vi "1 sample delay 8spc.vi"(8 "input valid":bool=TRUE, 10 "delay":u8, 11 "IQ in":T1(array[cluster])=[{"I"=0.0, "Q"=0.0, "overflow"=FALSE}, {"I"=0.0, "Q"=0.0, "overflow"=FALSE}, {"I"=0.0, "Q"=0.0, "overflow"=FALSE}, {"I"=0.0, "Q"=0.0, "overflow"=FALSE}, {"I"=0.0, "Q"=0.0, "overflow"=FALSE}, {"I"=0.0, "Q"=0.0, "overflow"=FALSE}, {"I"=0.0, "Q"=0.0, "overflow"=FALSE}, {"I"=0.0, "Q"=0.0, "overflow"=FALSE}]) -> (0 "output valid":bool, 3 "IQ out":T1(array[cluster]))   [LabVIEW 2021]
doc: "sum 2 IQ datas (I+I =>I ; Q+Q =>Q ; overflow or overflow or +overflow => overflow"
types:
  T1 = cluster{"I":fxp<+/-,18,1>, "Q":fxp<+/-,18,1>, "overflow":bool}[]
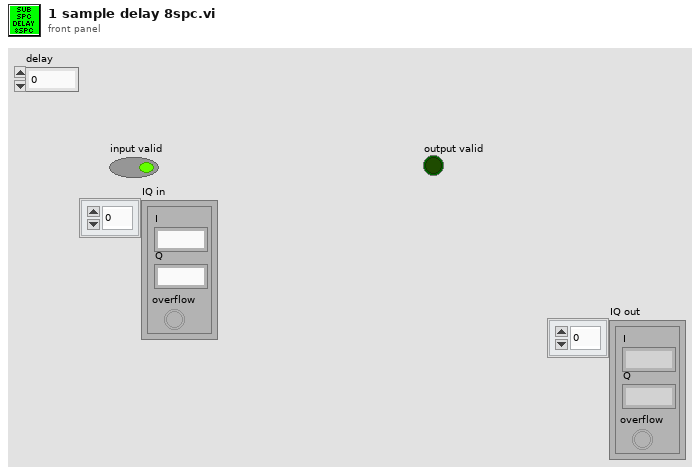
[diagram p1: front panel]
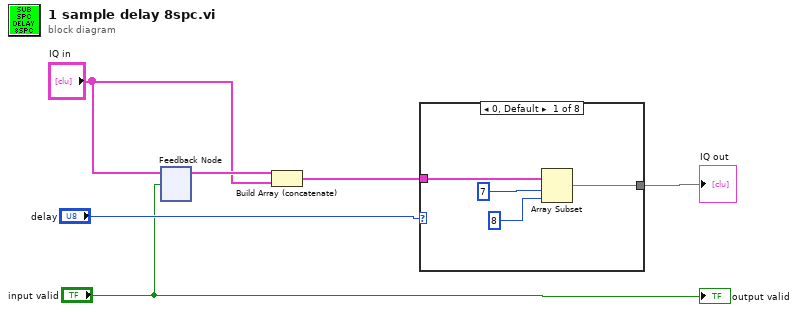
[diagram p0: block diagram]
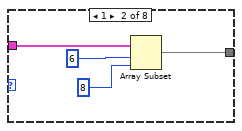
[diagram p2: hidden frame]
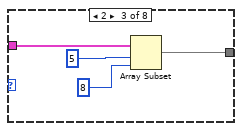
[diagram p3: hidden frame]
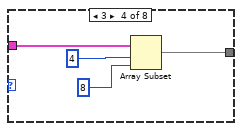
[diagram p4: hidden frame]
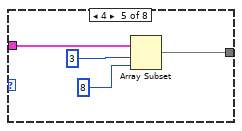
[diagram p5: hidden frame]
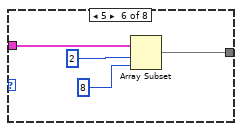
[diagram p6: hidden frame]
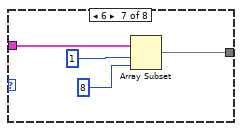
[diagram p7: hidden frame]
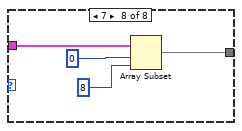
[diagram p8: hidden frame]
diagram:
  n1 = feedback #1() -> (w6:T1)  [unwired: 1 in]
  n2 = feedback-in #1("IQ in", "input valid") -> ()
  n3 = Build Array (concatenate)(w6, "IQ in") -> (w4:T1)
  n4 = case shown="0, Default" "delay" {
    tunnel: w4 -> [w10 w14 w18 w22 w26 w30 w34 w38]
    tunnel: [w8 w12 w16 w20 w24 w28 w32 w36] -> w3
    frame 0, Default {
      n5 = Array Subset(array=w10, index=7, length=8) -> (w8:T1)
    }
    frame 1 {
      n6 = Array Subset(array=w14, index=6, length=8) -> (w12:T1)
    }
    frame 2 {
      n7 = Array Subset(array=w18, index=5, length=8) -> (w16:T1)
    }
    frame 3 {
      n8 = Array Subset(array=w22, index=4, length=8) -> (w20:T1)
    }
    frame 4 {
      n9 = Array Subset(array=w26, index=3, length=8) -> (w24:T1)
    }
    frame 5 {
      n10 = Array Subset(array=w30, index=2, length=8) -> (w28:T1)
    }
    frame 6 {
      n11 = Array Subset(array=w34, index=1, length=8) -> (w32:T1)
    }
    frame 7 {
      n12 = Array Subset(array=w38, index=0, length=8) -> (w36:T1)
    }
  }
  "IQ out" <- w3
  "output valid" <- "input valid"
